vi "Agilent E4980 Read Measurement List Sweep.vi"() -> ()   [LabVIEW 2016]
doc: "This example shows how to perform a list sweep and read the measured values."
uses:
  <instrlib>/Agilent E4980/Agilent E4980.lvlib
panel:
  out "Primary Parameter":dbl
  out "Secondary Parameter":dbl
  in  "Sweep Point Array":dbl[](array[numeric])=[1000.0, 2000.0, 5000.0]
  in  "List Band Limit Array":dbl[](array[numeric])=[100.0, 200.0, 100.0, 200.0, 100.0, 200.0]
  in  "VISA resource name":refnum<visa-resource-name>
  # "(c) 2007-2015 National Instruments.  ALL RIGHTS RESERVED."
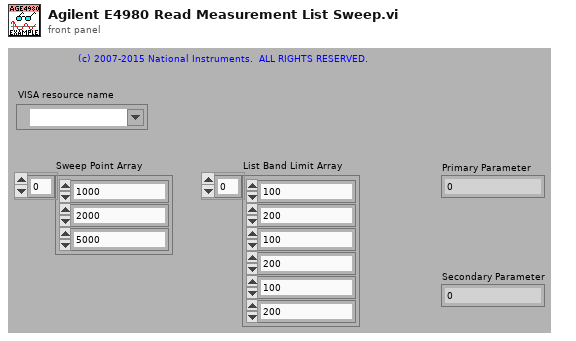
[diagram p1: front panel]
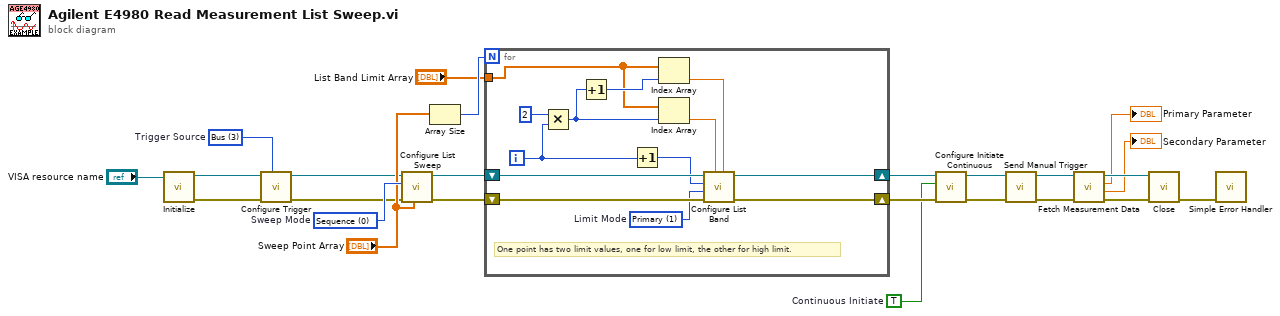
[diagram p0: block diagram]
diagram:
  w12 = TRUE  # Continuous Initiate
  w20 = u16 0 items=["Sequence", "Stepped"]  # Sweep Mode
  w21 = u16 3 items=["Internal", "Manual", "External", "Bus"]  # Trigger Source
  n1 = call <instrlib>:"Initialize.vi"("VISA resource name"="VISA resource name") -> ("error out"=w23:errorcluster, "VISA resource name out"=w24:refnum<visa-resource-name>)  [unwired: 9 in]
  n2 = call <instrlib>:"Configure Trigger.vi"("Trigger Source (0: Internal)"=w21, "error in (no error)"=w23, "VISA resource name"=w24) -> ("error out"=w1:errorcluster, "VISA resource name out"=w2:refnum<visa-resource-name>)  [unwired: 7 in]
  n3 = call <instrlib>:"Configure List Sweep.vi"("Sweep Point Array"="Sweep Point Array", "error in (no error)"=w1, "Sweep Mode (0: Sequence)"=w20, "VISA resource name"=w2) -> ("error out"=w16:errorcluster, "VISA resource name out"=w17:refnum<visa-resource-name>)  [unwired: 6 in]
  n4 = Array Size(array="Sweep Point Array") -> (size(s)=w18:i32)
  n5 = for {
    N: w18 -> [_]
    shift-right: [w35] -> w14
    shift-left: w17 -> [w37]
    shift-right: [w34] -> w13
    shift-left: w16 -> [w36]
    tunnel: "List Band Limit Array" -> [w25]
    i -> [w31]
    w33 = u16 1 items=["Off", "Primary", "Secondary"]  # Limit Mode
    # "One point has two limit values, one for low limit, the other for high limit."
    n6 = Multiply(x=2, y=w31) -> (x*y=w26:i32)
    n7 = Increment(x=w26) -> (x+1=w28:i32)
    n8 = Increment(x=w31) -> (x+1=w32:i32)
    n9 = Index Array(array=w25, index=w28) -> (element=w27:dbl)
    n10 = Index Array(array=w25, index=w26) -> (element=w29:dbl)
    n11 = call <instrlib>:"Configure List Band.vi"("High Limit (0)"=w27, "Low Limit (0)"=w29, "error in (no error)"=w36, "Limit Mode (0:Off)"=w33, "Point No. (1)"=w32, "VISA resource name"=w37) -> ("error out"=w34:errorcluster, "VISA resource name out"=w35:refnum<visa-resource-name>)  [unwired: 4 in]
  }
  n12 = call <instrlib>:"Configure Initiate Continuous.vi"("error in (no error)"=w13, "Continuous Initiate (F:Disable)"=w12, "VISA resource name"=w14) -> ("error out"=w10:errorcluster, "VISA resource name out"=w11:refnum<visa-resource-name>)  [unwired: 7 in]
  n13 = call <instrlib>:"Send Manual Trigger.vi"("error in (no error)"=w10, "VISA resource name"=w11) -> ("error out"=w8:errorcluster, "VISA resource name out"=w9:refnum<visa-resource-name>)  [unwired: 8 in]
  n14 = call <instrlib>:"Fetch Measurement Data.vi"("error in (no error)"=w8, "VISA resource name"=w9) -> ("error out"=w6:errorcluster, "Secondary Parameter"=→"Secondary Parameter":dbl, "Primary Parameter"=→"Primary Parameter":dbl, "VISA resource name out"=w7:refnum<visa-resource-name>)  [unwired: 5 in, 1 out]
  n15 = call <instrlib>:"Close.vi"("error in (no error)"=w6, "VISA resource name"=w7) -> ("error out"=w5:errorcluster)  [unwired: 9 in]
  n16 = call <vilib>:"Simple Error Handler.vi"("error in (no error)"=w5) -> ()  [unwired: 4 in, 5 out]
